vi "FATEK-Response Message Format.vi"(8 "error in":errorcluster, 11 "Response Data":string) -> (0 "error out":errorcluster, 3 "Read Response Message":T1={"Slave Station No"="01", "Command Code"=72, "Error Code"=0, "Response Data"=[]} {"Command Code" items=["Read multiple data of consecutive registers"=70, "Write to multiple consecutive registers"=71]})   [LabVIEW 2018]
uses:
  Data Def/FATEK-Read Response Message.ctl
  Data Def/FATEK-Command Code.ctl
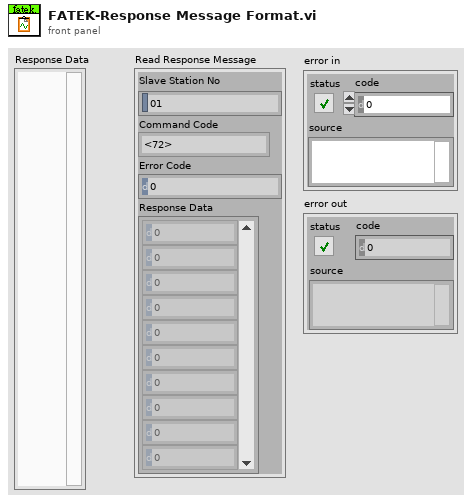
[diagram p1: front panel]
types:
  T1 = typedef "FATEK-Read Response Message.ctl" = cluster{"Slave Station No":string, "Command Code":T2, "Error Code":u8, "Response Data":i16[]}
  T2 = typedef "FATEK-Command Code.ctl" = u16
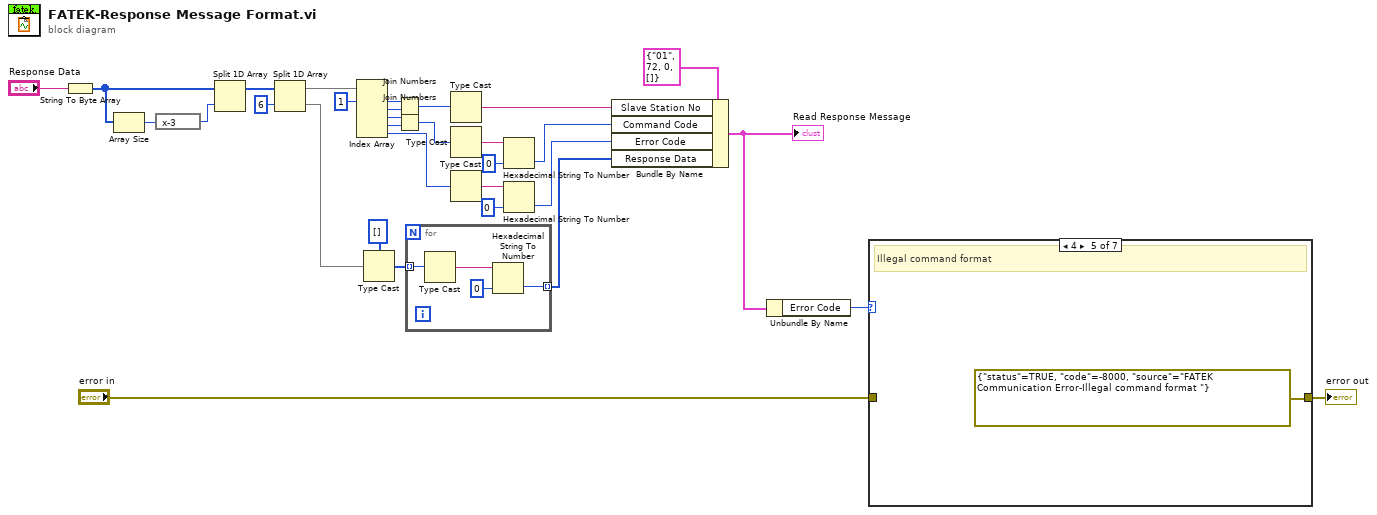
[diagram p0: block diagram]
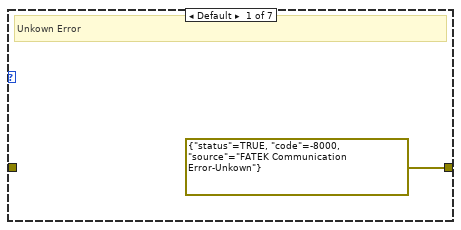
[diagram p2: hidden frame]
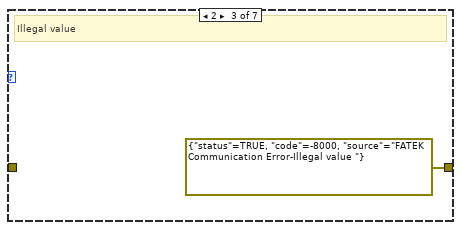
[diagram p4: hidden frame]
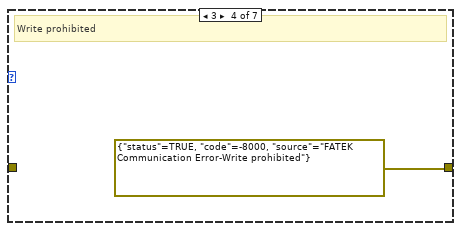
[diagram p5: hidden frame]
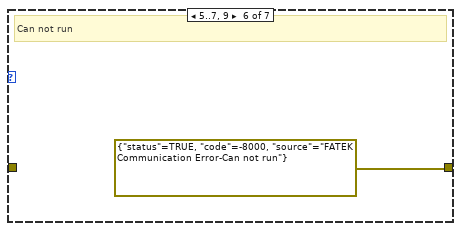
[diagram p6: hidden frame]
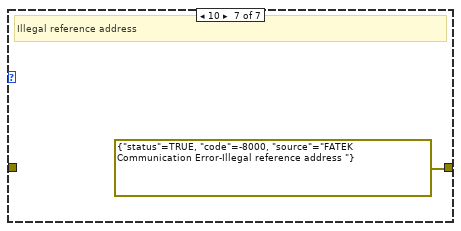
[diagram p7: hidden frame]
diagram:
  n1 = String To Byte Array(string="Response Data") -> (unsigned byte array=w13:u8[])
  n2 = Array Size(array=w13) -> (size(s)=w14:i32)
  n3 = expression code="x-3"(w14) -> (w12:i32)
  n4 = Split 1D Array(array=w13, index=w12) -> (first subarray=w11:u8[])  [unwired: 1 out]
  n5 = Split 1D Array(array=w11, index=6) -> (first subarray=w10:u8[], second subarray=w8:u8[])
  n6 = Index Array(array=w10, index #1=1 ("index")) -> (element #1=w29:u8, element #2=w28:u8, element #3=w23:u8, element #4=w24:u8, element #5=w18:u8)  [unwired: 4 in]
  n7 = Type Cast(type=u32[] [], x=w8) -> (*(type *) &x=w6:u32[])
  n8 = Join Numbers(hi=w29, lo=w28) -> ((hi.lo)=w27:u16)
  n9 = Join Numbers(hi=w23, lo=w24) -> ((hi.lo)=w22:u16)
  n10 = for {
    tunnel: w6 -> [w35] mode=indexing
    tunnel: [w32] -> w1 mode=indexing
    n11 = Type Cast(x=w35) -> (*(type *) &x=w34:string)  [unwired: 1 in]
    n12 = Hexadecimal String To Number(string=w34, default (0uL)=i16 0 ("default (0 U32)")) -> (number=w32:i16)  [unwired: 1 in, 1 out]
  }
  n13 = Type Cast(x=w27) -> (*(type *) &x=w25:string)  [unwired: 1 in]
  n14 = Type Cast(x=w22) -> (*(type *) &x=w19:string)  [unwired: 1 in]
  n15 = Type Cast(x=w18) -> (*(type *) &x=w16:string)  [unwired: 1 in]
  n16 = Hexadecimal String To Number(string=w19, default (0uL)=u16 0 ("default (0 U32)")) -> (number=w20:u16)  [unwired: 1 in, 1 out]
  n17 = Hexadecimal String To Number(string=w16, default (0uL)=u8 0 ("default (0 U32)")) -> (number=w15:u8)  [unwired: 1 in, 1 out]
  n18 = Bundle By Name(cluster=T1 {"Slave Station No"="01", "Command Code"=72, "Error Code"=0, "Response Data"=[]} ("Read Response Message"), "Slave Station No"=w25, "Command Code"=w20, "Error Code"=w15, "Response Data"=w1) -> (w5:T1)
  "Read Response Message" <- w5
  n19 = Unbundle By Name(w5) -> ("Error Code"=w4:u8)
  n20 = case shown="4" w4 {
    tunnel: "error in" -> [_ w37 _ _ _ _ _]
    tunnel: [errorcluster {"status"=TRUE, "code"=-8000, "source"="FATEK Communication Error-Unkown"} ("error in") w37 errorcluster {"status"=TRUE, "code"=-8000, "source"="FATEK Communication Error-Illegal value "} ("error in") errorcluster {"status"=TRUE, "code"=-8000, "source"="FATEK Communication Error-Write prohibited"} ("error in") errorcluster {"status"=TRUE, "code"=-8000, "source"="FATEK Communication Error-Illegal command format "} ("error in") errorcluster {"status"=TRUE, "code"=-8000, "source"="FATEK Communication Error-Can not run"} ("error in") errorcluster {"status"=TRUE, "code"=-8000, "source"="FATEK Communication Error-Illegal reference address "} ("error in")] -> w2
    frame Default {
      # "Unkown Error"
    }
    frame 0 {
      # "No Error"
    }
    frame 2 {
      # "Illegal value"
    }
    frame 3 {
      # "Write prohibited"
    }
    frame 4 {
      # "Illegal command format"
    }
    frame 5..7, 9 {
      # "Can not run"
    }
    frame 10 {
      # "Illegal reference address"
    }
  }
  "error out" <- w2
